vi "SubPanel.vi"() -> ()   [LabVIEW 2016, in "test_ValueSignal.lvlib"]
uses:
  test_ValueSignal.lvlib
  main/apis/Setup/GetVI/GetVIByPath.vi
  main/apis/Stimulus/ValueSignal/ValueSignalByPathString.vi
  main/apis/Assert/AssertControlValue/Equal.vi
  <vilib>/addons/_JKI Toolkits/Caraya/classes/Test/Test.lvclass
  main/apis/Setup/GetVI/GetVI.lvlib
  main/apis/Assert/AssertControlValue/AssertControlValue.lvlib
panel:
  out "error out":errorcluster
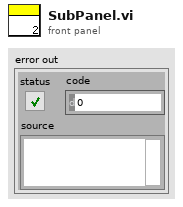
[diagram p1: front panel]
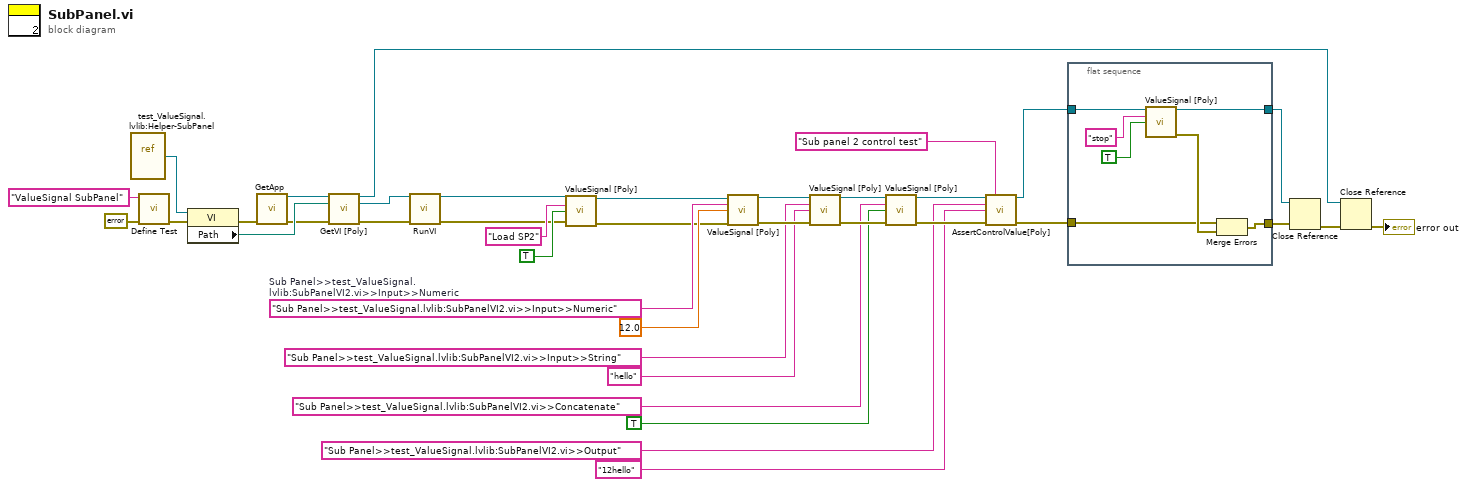
[diagram p0: block diagram]
diagram:
  w20 = "Sub Panel>>test_ValueSignal.lvlib:SubPanelVI2.vi>>Input>>Numeric"  # Sub Panel>>test_ValueSignal.lvlib:SubPanelVI2.vi>>Input>>Numeric
  n1 = vi-ref "test_ValueSignal.lvlib:Helper-SubPanel.vi"() -> (w9:refnum<vi>)
  n2 = call <vilib>:"Define Test.vi"("error in (no error)"=errorcluster {"status"=FALSE, "code"=0, "source"=""}, "Label (VI Title)"="ValueSignal SubPanel") -> ("error out"=w10:errorcluster)  [unwired: 9 in]
  n3 = property on="Property Node" class="VI"(reference=w9, error in=w10) -> (error out=w37:errorcluster, "Path"=w36:path)  [unwired: 1 out]
  n4 = call "GetApp.vi"("error in (no error)"=w37) -> ("Application Ref"=w38:refnum<vi>, "error out"=w35:errorcluster)  [unwired: 13 in]
  n5 = call-poly "GetVI [Poly].vi"("Application Ref in"=w38, "VI Path"=w36, "error in (no error)"=w35) -> ("Application Ref out"=w34:refnum<vi>, "VI Reference"=w16:refnum<vi>, "error out"=w14:errorcluster)  [unwired: 10 in]
  n6 = call "RunVI.vi"("VI Reference In"=w16, "error in"=w14) -> ("VI Reference Out"=w15:refnum<vi>, "error out"=w13:errorcluster)  [unwired: 12 in]
  n7 = call-poly "ValueSignal [Poly].vi"("VI Reference In"=w15, "Control Name"="Load SP2" ("Class Name"), "Value (Signaling)"=TRUE, "error in"=w13) -> ("VI Reference Out"=w17:refnum<vi>, "error out"=w18:errorcluster)  [unwired: 10 in]
  n8 = call-poly "ValueSignal [Poly].vi"("VI Reference In"=w17, "Control Name"=w20, "Value (Signaling)"=12.0, "error in"=w18) -> ("VI Reference Out"=w26:refnum<vi>, "error out"=w27:errorcluster)  [unwired: 10 in]
  n9 = call-poly "ValueSignal [Poly].vi"("VI Reference In"=w26, "Control Name"="Sub Panel>>test_ValueSignal.lvlib:SubPanelVI2.vi>>Input>>String", "Value (Signaling)"="hello" ("Control Name"), "error in"=w27) -> ("VI Reference Out"=w23:refnum<vi>, "error out"=w24:errorcluster)  [unwired: 10 in]
  n10 = call-poly "ValueSignal [Poly].vi"("VI Reference In"=w23, "Control Name"="Sub Panel>>test_ValueSignal.lvlib:SubPanelVI2.vi>>Concatenate", "Value (Signaling)"=TRUE, "error in"=w24) -> ("VI Reference Out"=w7:refnum<vi>, "error out"=w5:errorcluster)  [unwired: 10 in]
  n11 = call-poly "AssertControlValue[Poly].vi"("VI Reference In"=w7, "Label"="Sub panel 2 control test" ("Label (VI Title)"), "Control Name"="Sub Panel>>test_ValueSignal.lvlib:SubPanelVI2.vi>>Output", "Control Value"="12hello" ("Control Name"), "Error In"=w5) -> ("VI Reference Out"=w6:refnum<vi>, "Error Out"=w4:errorcluster)  [unwired: 9 in]
  n12 = flat-sequence {
    tunnel: [w41] -> w32
    tunnel: [w42] -> w31
    tunnel: w6 -> [w40]
    tunnel: w4 -> [w39]
    frame #0 {
      n13 = call-poly "ValueSignal [Poly].vi"("VI Reference In"=w40, "Control Name"="stop" ("Class Name"), "Value (Signaling)"=TRUE) -> ("VI Reference Out"=w42:refnum<vi>, "error out"=w43:errorcluster)  [unwired: 11 in]
      n14 = Merge Errors(w39, w43) -> (w41:errorcluster)
    }
  }
  n15 = Close Reference(reference=w31, error in (no error)=w32) -> (error out=w33:errorcluster)
  n16 = Close Reference(reference=w34, error in (no error)=w33) -> (error out=→"error out":errorcluster)
